vi "add to table.vi"(9 "value":dbl, 10 "key":string, 11 "lookup table":T1(array[cluster])) -> (3 "lookup table out":T1(array[cluster]))   [LabVIEW 2013]
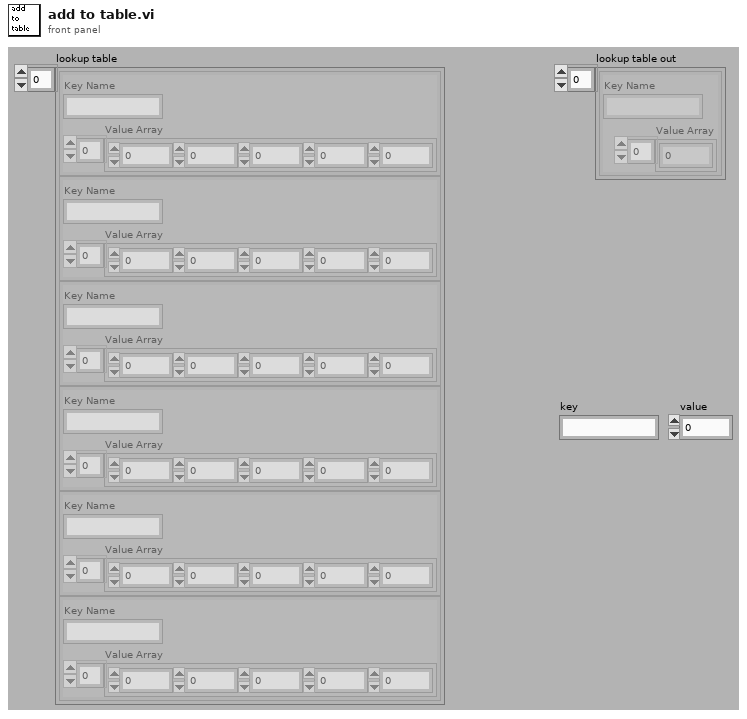
[diagram p1: front panel]
types:
  T1 = cluster{"Key Name":string, "Value Array":dbl[]}[]
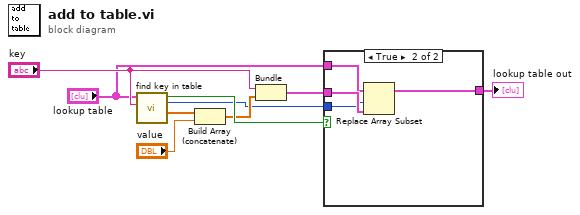
[diagram p0: block diagram]
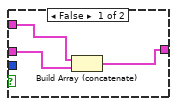
[diagram p2: hidden frame]
diagram:
  n1 = call "find key in table.vi"("key"="key", "lookup table"="lookup table") -> ("Value Array"=w9:dbl[], "location"=w3:i32, "found"=w7:bool)  [unwired: 7 in]
  n2 = Build Array (concatenate)(w9, "value") -> (w5:dbl[])
  n3 = Bundle("key"="key", w5) -> (w4:cluster{"key":string, dbl[]})  [unwired: 1 in]
  n4 = case shown="True" w7 {
    tunnel: w4 -> [w11 w16]
    tunnel: w3 -> [_ w15]
    tunnel: "lookup table" -> [w12 w14]
    tunnel: [w10 w13] -> w1
    frame False {
      n5 = Build Array (concatenate)(w12, w11) -> (w10:cluster{"key":string, "Value Array":dbl[]}[])
    }
    frame True {
      n6 = Replace Array Subset(array=w14, new element=w16, index=w15) -> (w13:T1)
    }
  }
  "lookup table out" <- w1
